vi "SOC_FM Main.vi"() -> ()   [LabVIEW 2015]
doc: "This sample project is built upon the standard state machine template and shows how you could create an application that acquires, analyzes, and presents data. It includes functionality for presenting configuration dialogs, preserving settings between executions, loading and saving data, as well as exporting graph images and text files.\n\nIt is most appropriate for data that is acquired instantly as it does not allow for screen updates mid acquisition nor does it allow for continuous streaming to disk."
uses:
  controls/SOC_FM State.ctl
  controls/SOC_FM Data.ctl
  controls/SOC_FM UI References.ctl
  controls/SOC_FM Graph Data.ctl
  <vilib>/Utility/miscctls.llb/LVAnnotationListTypeDef.ctl
  <vilib>/Utility/miscctls.llb/LVCursorListTypeDef.ctl
  controls/SOC_FM HW Configuration.ctl
  controls/SOC_FM Simulated Signal Type.ctl
  controls/SOC_FM Analysis Configuration.ctl
  controls/SOC_FM New Data Behavior.ctl
  PPL/AbstractCalcLib.lvlibp/AbstractCalc/AbstractCalc.lvclass
  subVIs/SOC_FM Settings Dialog.vi
panel:
  in  "Settings":bool
  in  "Snapshot":bool
  in  "Analyze":bool
  in  "Clear":bool
  in  "Exit":bool
  in  "Acquire":bool
  in  "Export":bool
  in  "Save Data":bool
  in  "Load Data":bool
  out "Graph":waveform(dbl)[](graph)
  out "Status Bar":string
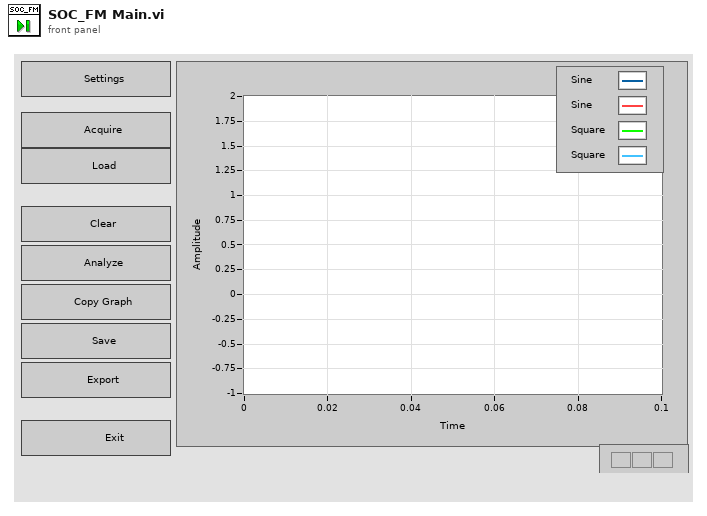
[diagram p1: front panel]
types:
  T1 = typedef "SOC_FM Data.ctl" = cluster{"UI References":T2, "Graph Data":T3, "User Specified":cluster{"Hardware Configuration":T6, "Analysis Configuration":T8, "New Data Behavior":T9, "Calc PPL Path":path, "Calc Plugin Class Qualified Name":string, "Calc Configuration String":string}, "AbstractCalc":refnum<class "AbstractCalc.lvclass">}
  T2 = typedef "SOC_FM UI References.ctl" = cluster{"Exit Ref":refnum<vi>, "Save Ref":refnum<vi>, "Open Ref":refnum<vi>, "Export Ref":refnum<vi>, "Acquire Ref":refnum<vi>, "Configure Ref":refnum<vi>, "Graph Ref":refnum<vi>, "Clear Ref":refnum<vi>, "Analyze Ref":refnum<vi>, "Status Ref":refnum<vi>, "Snapshot Ref":refnum<vi>}
  T3 = typedef "SOC_FM Graph Data.ctl" = cluster{"Data":waveform(dbl)[], "Annotation List":T4, "Cursor List":T5, "Analysis Data":waveform(dbl)[]}
  T4 = typedef "LVAnnotationListTypeDef.ctl" = cluster{"Name":string, "Color":u32, "Style":u8, "Point Style":u8, "Name Visible":bool, "Allow Drag":bool, "Annotation Mode":u32, "Plot":i32, "Index":i32, "Position":cluster{"X":dbl, "Y":dbl}, "X Scale":u32, "Y Scale":u32, "Show Arrow":bool, "Lock Name":bool, "Plot Area":i32, "Label Offset":cluster{"X":dbl, "Y":dbl}}[]
  T5 = typedef "LVCursorListTypeDef.ctl" = cluster{"Name":string, "Color":u32, "Style":u8, "Point Style":u8, "Name Visible":bool, "Allow Drag":bool, "Cursor Mode":u32, "Plot":i32, "Index":i32, "Position":cluster{"X":dbl, "Y":dbl}, "X Scale":u32, "Y Scale":u32, "Watch Plots":i32[], "Watch All Plots":bool, "Plot Area":i32, "Label Offset":cluster{"X":dbl, "Y":dbl}}[]
  T6 = typedef "SOC_FM HW Configuration.ctl" = cluster{"HW Refnum <Replace Me>":string, "Signal Type <Replace Me>":T7}
  T7 = typedef "SOC_FM Simulated Signal Type.ctl" = enum16{"Sine Wave", "Square Wave"}
  T8 = typedef "SOC_FM Analysis Configuration.ctl" = cluster{"Statistics":bool}
  T9 = typedef "SOC_FM New Data Behavior.ctl" = enum16{"Replace", "Overlay", "Append"}
  T10 = typedef "SOC_FM State.ctl" = enum16{"Initialize", "Wait for Event", "Update UI", "Configure", "Acquire", "Load Data", "Save Data", "Clear Data", "Export Data", "Analyze", "Copy Graph", "Exit"}
  T11 = cluster{"Hardware Configuration":T6, "Analysis Configuration":T8, "New Data Behavior":T9, "Calc PPL Path":path, "Calc Plugin Class Qualified Name":string, "Calc Configuration String":string}
  T12 = typedef "SOC_FM User Specified Data.ctl" = cluster{"Hardware Configuration":T6, "Analysis Configuration":T8, "New Data Behavior":T9, "Calc PPL Path":path, "Calc Plugin Class Qualified Name":string, "Calc Configuration String":string}
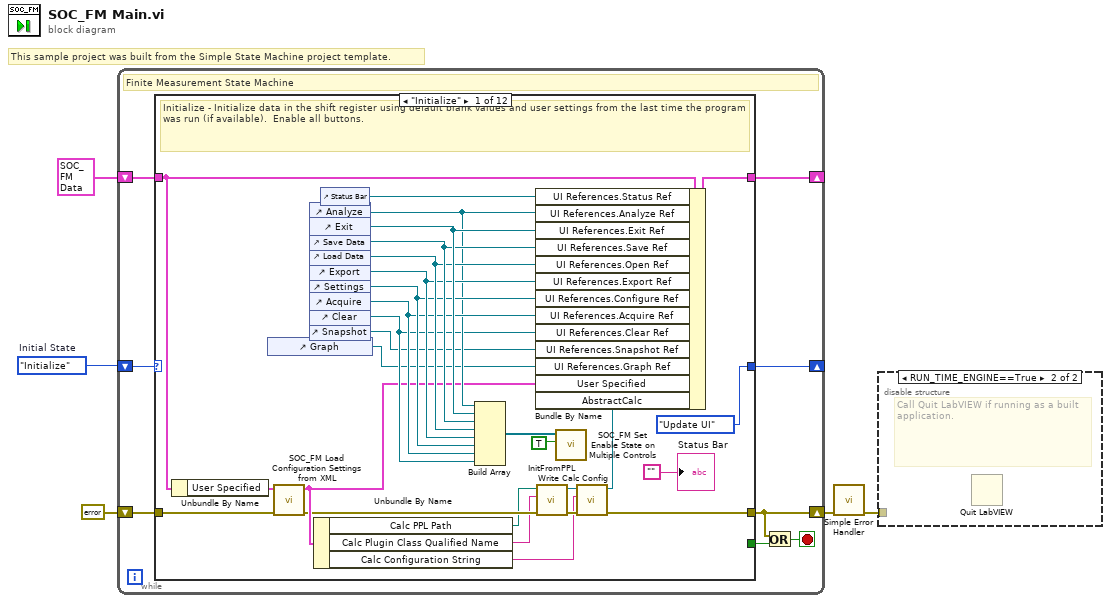
[diagram p0: block diagram]
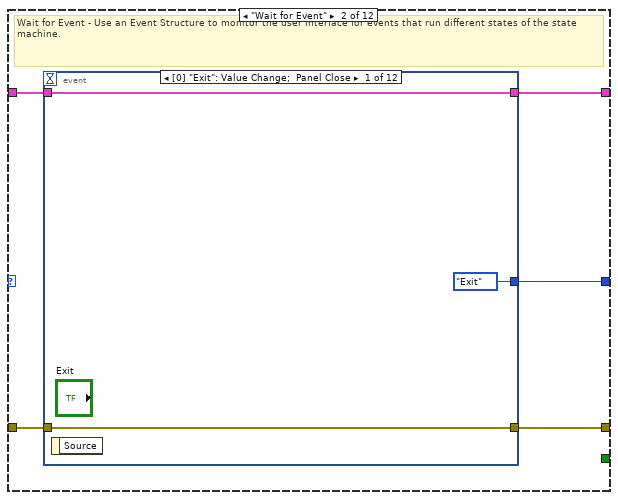
[diagram p3: hidden frame]
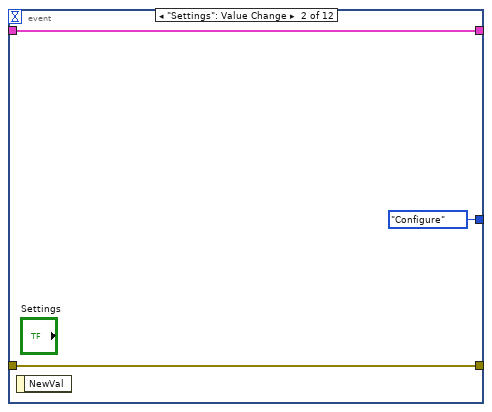
[diagram p4: hidden frame]
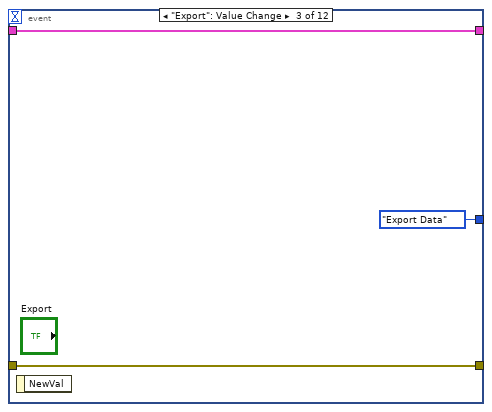
[diagram p5: hidden frame]
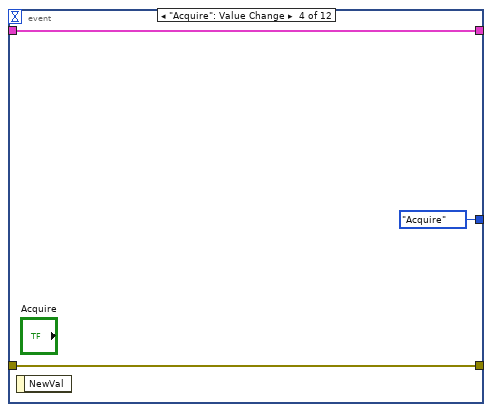
[diagram p6: hidden frame]
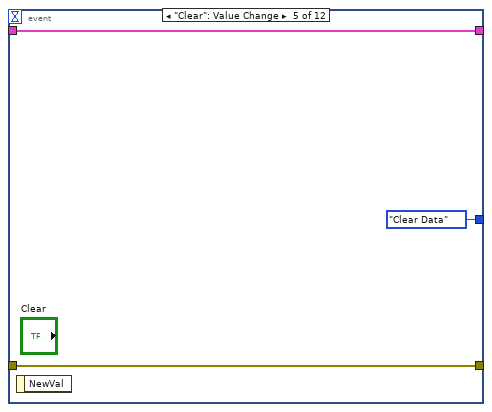
[diagram p7: hidden frame]
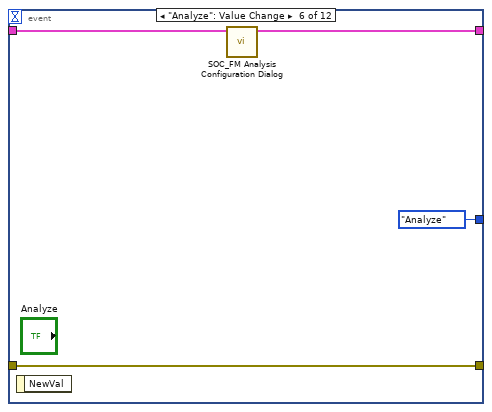
[diagram p8: hidden frame]
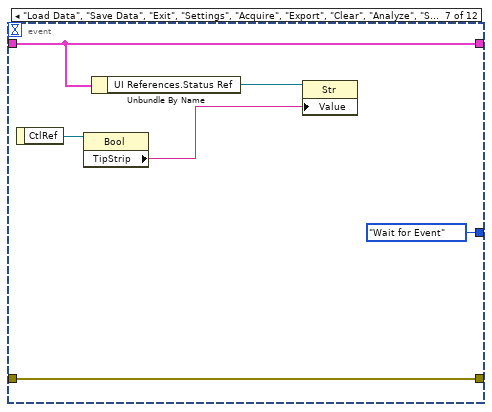
[diagram p9: hidden frame]
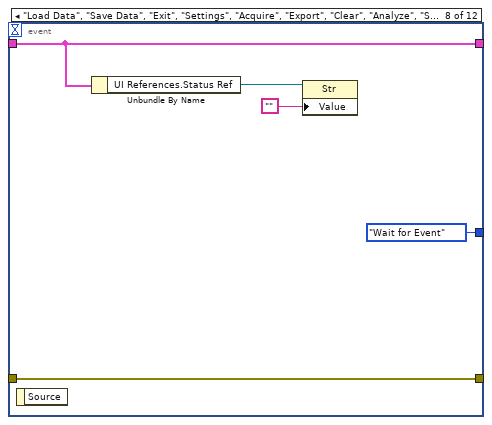
[diagram p10: hidden frame]
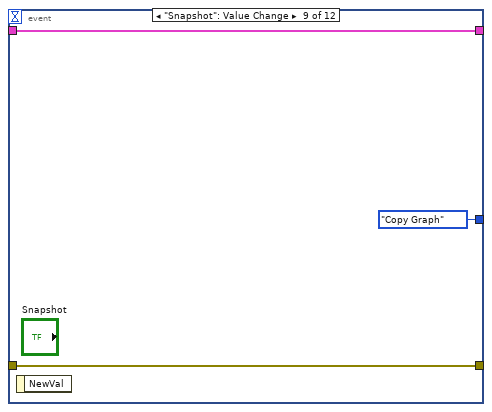
[diagram p11: hidden frame]
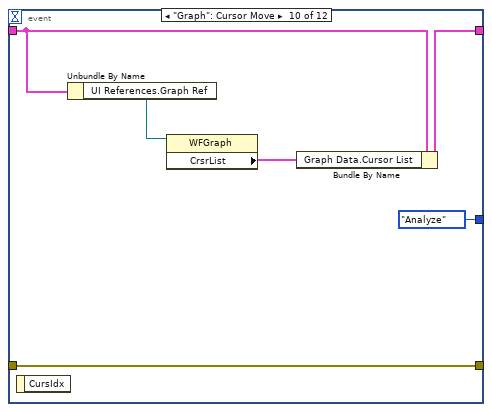
[diagram p12: hidden frame]
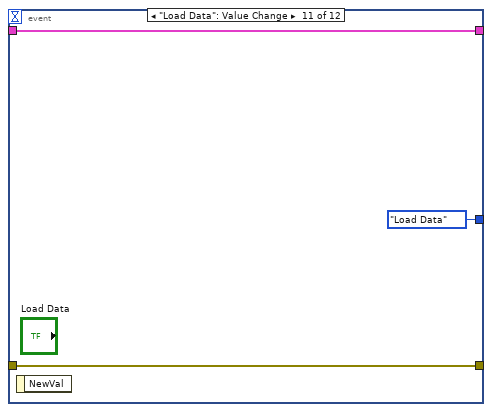
[diagram p13: hidden frame]
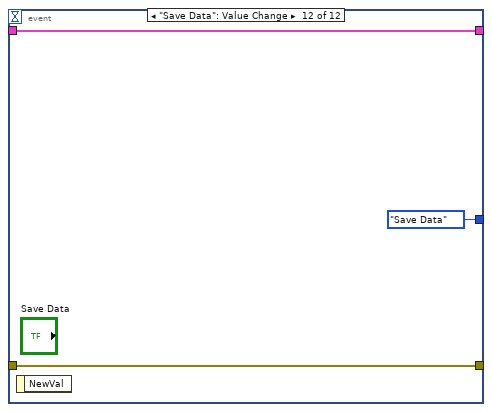
[diagram p14: hidden frame]
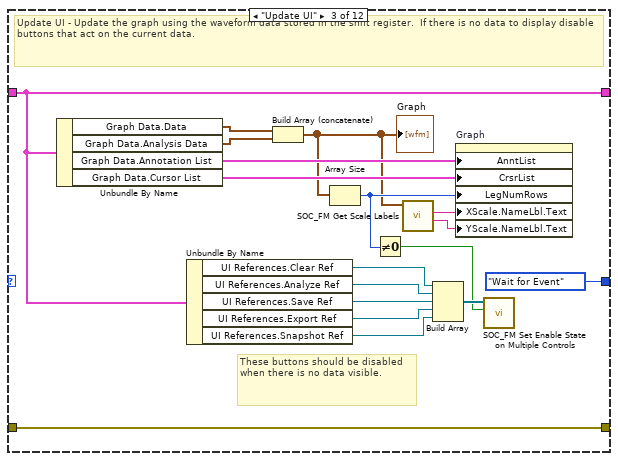
[diagram p15: hidden frame]
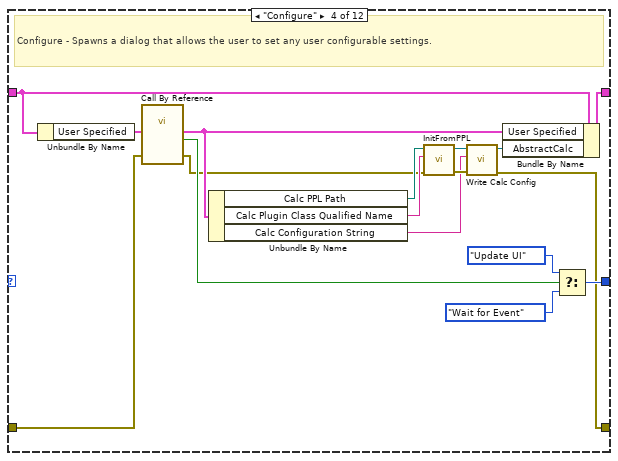
[diagram p16: hidden frame]
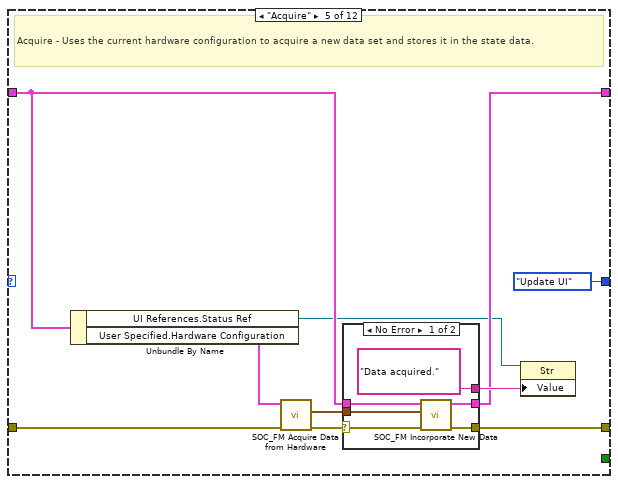
[diagram p17: hidden frame]
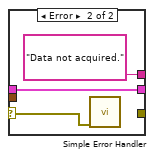
[diagram p18: hidden frame]
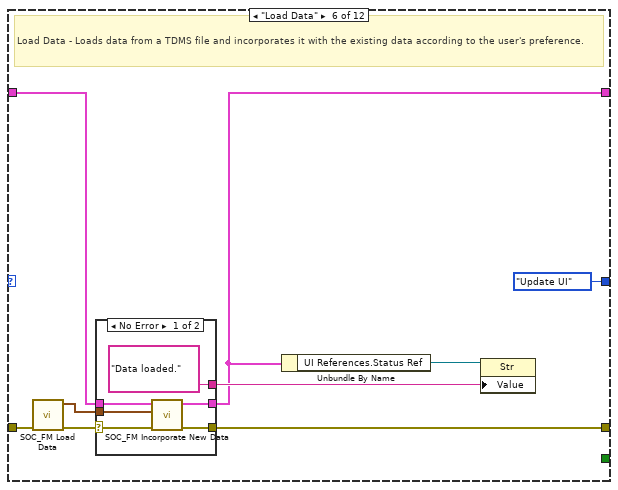
[diagram p19: hidden frame]
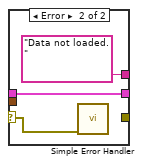
[diagram p20: hidden frame]
diagram:
  w5 = SOC_FM_State."Initialize"  # Initial State
  # "This sample project was built from the Simple State Machine project template."
  n1 = while {
    shift-right: [w12] -> _
    shift-left: w5 -> [w13]
    shift-right: [w10] -> _
    shift-left: T1 {"UI References"={"Exit Ref"=refnum, "Save Ref"=refnum, "Open Ref"=refnum, "Export Ref"=refnum, "Acquire Ref"=refnum, "Configure Ref"=refnum, "Graph Ref"=refnum, "Clear Ref"=refnum, "Analyze Ref"=refnum, "Status Ref"=refnum, "Snapshot Ref"=refnum}, "Graph Data"={"Data"=[], "Annotation List"=[], "Cursor List"=[], "Analysis Data"=[]}, "User Specified"={"Hardware Configuration"={"HW Refnum <Replace Me>"="", "Signal Type <Replace Me>"=enum."Sine Wave"}, "Analysis Configuration"={"Statistics"=TRUE}, "New Data Behavior"=enum."Replace", "Calc PPL Path"=path "", "Calc Plugin Class Qualified Name"="", "Calc Configuration String"=""}, "AbstractCalc"=refnum} ("Data") -> [w11]
    shift-right: [w6] -> w3
    shift-left: errorcluster {"status"=FALSE, "code"=0, "source"=""} ("error constant") -> [w9]
    stop <- w7 stop-if-true
    # "Finite Measurement State Machine"
    n2 = case shown="\"Initialize\"" w13 {
      tunnel: [SOC_FM_State."Update UI" ("Next State") w46 SOC_FM_State."Wait for Event" ("(Value Not Used)") w121 SOC_FM_State."Update UI" ("Next State") SOC_FM_State."Update UI" ("(Value Not Used)") SOC_FM_State."Wait for Event" ("(Value Not Used)") SOC_FM_State."Wait for Event" ("(Value Not Used)") SOC_FM_State."Update UI" ("(Value Not Used)") SOC_FM_State."Update UI" ("(Value Not Used)") SOC_FM_State."Wait for Event" ("(Value Not Used)") w212] -> w12
      tunnel: [_ _ _ _ _ _ _ _ _ _ _ w211] -> w8
      tunnel: w11 -> [w32 w45 w106 w126 w132 w154 w167 w179 w190 w199 w203 w209]
      tunnel: [w40 w44 w106 w125 w131 w148 w167 w179 w189 w199 w203 w209] -> w10
      tunnel: w9 -> [w30 w43 w109 w124 w134 w153 w169 w182 w192 w196 w202 w206]
      tunnel: [w19 w42 w109 w110 w127 w152 w165 w176 w192 w193 w201 w205] -> w6
      frame "Initialize" {
        # "Initialize - Initialize data in the shift register using default blank values and user settings from the last time the program was run (if available).  Enable all buttons."
        n3 = Unbundle By Name(w32) -> ("User Specified"=w31:T11)
        n4 = control-ref of="Graph"() -> (w23:refnum<vi>)
        n5 = call "SOC_FM Load Configuration Settings from XML.vi"("error in (no error)"=w30, "User Specified"=w31) -> ("error out"=w21:errorcluster, "User Specified 2"=w22:T12)  [unwired: 8 in]
        n6 = control-ref of="Analyze"() -> (w29:refnum<vi>)
        n7 = control-ref of="Exit"() -> (w39:refnum<vi>)
        n8 = control-ref of="Save Data"() -> (w38:refnum<vi>)
        n9 = control-ref of="Load Data"() -> (w37:refnum<vi>)
        n10 = control-ref of="Export"() -> (w36:refnum<vi>)
        n11 = control-ref of="Settings"() -> (w35:refnum<vi>)
        n12 = control-ref of="Acquire"() -> (w34:refnum<vi>)
        n13 = control-ref of="Clear"() -> (w27:refnum<vi>)
        n14 = control-ref of="Snapshot"() -> (w24:refnum<vi>)
        n15 = Unbundle By Name(w22) -> ("Calc PPL Path"=w14:path, "Calc Plugin Class Qualified Name"=w15:string, "Calc Configuration String"=w17:string)
        n16 = control-ref of="Status Bar"() -> (w28:refnum<vi>)
        n17 = Build Array(w29, w39, w38, w37, w36, w35, w34, w27) -> (w33:refnum<vi>[])
        n18 = call "InitFromPPL.vi"("error in (no error)"=w21, "qualified name"=w15, "packed library path"=w14) -> ("error out"=w20:errorcluster, "AbstractCalc out"=w16:refnum<class "AbstractCalc.lvclass">)  [unwired: 7 in]
        n19 = call "SOC_FM Set Enable State on Multiple Controls.vi"("Enable?"=TRUE, "Controls"=w33) -> ()  [unwired: 10 in]
        n20 = call-dynamic "Write Calc Config.vi"("error in (no error)"=w20, "Config String"=w17, "AbstractCalc in"=w16) -> ("error out"=w19:errorcluster, "AbstractCalc out"=w18:refnum<class "AbstractCalc.lvclass">)  [unwired: 7 in]
        n21 = Bundle By Name(cluster=w32, "UI References.Status Ref"=w28, "UI References.Analyze Ref"=w29, "UI References.Exit Ref"=w39, "UI References.Save Ref"=w38, "UI References.Open Ref"=w37, "UI References.Export Ref"=w36, "UI References.Configure Ref"=w35, "UI References.Acquire Ref"=w34, "UI References.Clear Ref"=w27, "UI References.Snapshot Ref"=w24, "UI References.Graph Ref"=w23, "User Specified"=w22, "AbstractCalc"=w18) -> (w40:T1)
        "Status Bar" <- "" ("Status Bar")
      }
      frame "Wait for Event" {
        # "Wait for Event - Use an Event Structure to monitor the user interface for events that run different states of the state machine."
        n22 = event shown="[0] \"Exit\": Value Change;  Panel Close" {
          selector: _ -> [_ _ _ _ _ _ _ _ _ _ _ _]
          dyn-events: _ -> [_ _ _ _ _ _ _ _ _ _ _ _]
          timeout: _ -> [_ _ _ _ _ _ _ _ _ _ _ _]
          tunnel: [SOC_FM_State."Exit" ("Next State") SOC_FM_State."Configure" ("Next State") SOC_FM_State."Export Data" ("Next State") SOC_FM_State."Acquire" ("Next State") SOC_FM_State."Clear Data" ("Next State") SOC_FM_State."Analyze" ("Next State") SOC_FM_State."Wait for Event" ("Next State") SOC_FM_State."Wait for Event" ("Next State") SOC_FM_State."Copy Graph" ("Next State") SOC_FM_State."Analyze" ("Next State") SOC_FM_State."Load Data" ("Next State") SOC_FM_State."Save Data" ("Next State")] -> w46
          tunnel: w45 -> [w48 w52 w55 w58 w61 w63 w69 w75 w79 w80 w87 w90]
          tunnel: [w48 w52 w55 w58 w61 w62 w69 w75 w79 w83 w87 w90] -> w44
          tunnel: w43 -> [w47 w51 w54 w57 w60 w65 w71 w76 w78 w85 w86 w89]
          tunnel: [w47 w51 w54 w57 w60 w65 w71 w76 w78 w85 w86 w89] -> w42
          event "Exit": Value Change; Panel Close {
            n23 = event-data() -> ()  [unwired: 1 in, 1 out]
          }
          event "Settings": Value Change {
            n24 = event-data() -> ()  [unwired: 1 in, 1 out]
          }
          event "Export": Value Change {
            n25 = event-data() -> ()  [unwired: 1 in, 1 out]
          }
          event "Acquire": Value Change {
            n26 = event-data() -> ()  [unwired: 1 in, 1 out]
          }
          event "Clear": Value Change {
            n27 = event-data() -> ()  [unwired: 1 in, 1 out]
          }
          event "Analyze": Value Change {
            n28 = event-data() -> ()  [unwired: 1 in, 1 out]
            n29 = call "SOC_FM Analysis Configuration Dialog.vi"("Data"=w63) -> ("Data 2"=w62:T1)  [unwired: 10 in]
          }
          event "Load Data", "Save Data", "Exit", "Settings", "Acquire", "Export", "Clear", "Analyze", "Snapshot": Mouse Enter {
            n30 = event-data() -> ("CtlRef"=w70:refnum<vi>)  [unwired: 1 in]
            n31 = property class="Bool"(reference=w70) -> ("TipStrip"=w67:string)  [unwired: 1 in, 2 out]
            n32 = Unbundle By Name(w69) -> ("UI References.Status Ref"=w68:refnum<vi>)
            n33 = property class="Str"(reference=w68, "Value"=w67) -> ()  [unwired: 1 in, 2 out]
          }
          event "Load Data", "Save Data", "Exit", "Settings", "Acquire", "Export", "Clear", "Analyze", "Snapshot": Mouse Leave {
            n34 = event-data() -> ()  [unwired: 1 in, 1 out]
            n35 = Unbundle By Name(w75) -> ("UI References.Status Ref"=w74:refnum<vi>)
            n36 = property class="Str"(reference=w74, "Value"="") -> ()  [unwired: 1 in, 2 out]
          }
          event "Snapshot": Value Change {
            n37 = event-data() -> ()  [unwired: 1 in, 1 out]
          }
          event "Graph": Cursor Move {
            n38 = event-data() -> ()  [unwired: 1 in, 1 out]
            n39 = Unbundle By Name(w80) -> ("UI References.Graph Ref"=w82:refnum<vi>)
            n40 = property class="WFGraph"(reference=w82) -> ("CrsrList"=w81:T5)  [unwired: 1 in, 2 out]
            n41 = Bundle By Name(cluster=w80, "Graph Data.Cursor List"=w81) -> (w83:T1)
          }
          event "Load Data": Value Change {
            n42 = event-data() -> ()  [unwired: 1 in, 1 out]
          }
          event "Save Data": Value Change {
            n43 = event-data() -> ()  [unwired: 1 in, 1 out]
          }
        }
      }
      frame "Update UI" {
        # "These buttons should be disabled when there is no data visible."
        # "Update UI - Update the graph using the waveform data stored in the shift register.  If there is no data to display disable buttons that act on the current data."
        n44 = Unbundle By Name(w106) -> ("Graph Data.Data"=w102:waveform(dbl)[], "Graph Data.Analysis Data"=w92:waveform(dbl)[], "Graph Data.Annotation List"=w107:T4, "Graph Data.Cursor List"=w103:T5)
        n45 = Unbundle By Name(w106) -> ("UI References.Clear Ref"=w98:refnum<vi>, "UI References.Analyze Ref"=w97:refnum<vi>, "UI References.Save Ref"=w105:refnum<vi>, "UI References.Export Ref"=w95:refnum<vi>, "UI References.Snapshot Ref"=w96:refnum<vi>)
        n46 = Build Array (concatenate)(w102, w92) -> (w100:waveform(dbl)[])
        "Graph" <- w100
        n47 = Array Size(array=w100) -> (size(s)=w101:i32)
        n48 = Not Equal To 0?(x=w101) -> (x != 0?=w99:bool)
        n49 = call "SOC_FM Get Scale Labels.vi"("Array of Waveforms"=w100) -> ("Y Scale Label Text"=w93:string, "X Scale Label Text"=w94:string)  [unwired: 9 in]
        n50 = Build Array(w98, w97, w105, w95, w96) -> (w104:refnum<vi>[])
        n51 = property on="Graph" class="WFGraph (strict)"("AnntList"=w107, "CrsrList"=w103, "LegNumRows"=w101, "XScale.NameLbl.Text"=w94, "YScale.NameLbl.Text"=w93) -> ()  [unwired: 2 in, 2 out]
        n52 = call "SOC_FM Set Enable State on Multiple Controls.vi"("Enable?"=w99, "Controls"=w104) -> ()  [unwired: 10 in]
      }
      frame "Configure" {
        # "Configure - Spawns a dialog that allows the user to set any user configurable settings."
        n53 = Unbundle By Name(w126) -> ("User Specified"=w119:T11)
        n54 = call-by-ref "?"("error in (no error)"=w124, "User Specified"=w119) -> ("error out"=w111:errorcluster, "UI Refresh Needed?"=w123:bool, "User Specified 2"=w117:T12)  [unwired: 9 in, 2 out]
        n55 = Unbundle By Name(w117) -> ("Calc PPL Path"=w114:path, "Calc Plugin Class Qualified Name"=w112:string, "Calc Configuration String"=w113:string)
        n56 = call "InitFromPPL.vi"("error in (no error)"=w111, "qualified name"=w112, "packed library path"=w114) -> ("error out"=w116:errorcluster, "AbstractCalc out"=w118:refnum<class "AbstractCalc.lvclass">)  [unwired: 7 in]
        n57 = call-dynamic "Write Calc Config.vi"("error in (no error)"=w116, "Config String"=w113, "AbstractCalc in"=w118) -> ("error out"=w110:errorcluster, "AbstractCalc out"=w115:refnum<class "AbstractCalc.lvclass">)  [unwired: 7 in]
        n58 = Bundle By Name(cluster=w126, "User Specified"=w117, "AbstractCalc"=w115) -> (w125:T1)
        n59 = Select(t=SOC_FM_State."Update UI" ("Next State if true"), s=w123, f=SOC_FM_State."Wait for Event" ("Next State if false")) -> (s? t:f=w121:T10)
      }
      frame "Acquire" {
        # "Acquire - Uses the current hardware configuration to acquire a new data set and stores it in the state data."
        n60 = Unbundle By Name(w132) -> ("UI References.Status Ref"=w128:refnum<vi>, "User Specified.Hardware Configuration"=w135:T6)
        n61 = call "SOC_FM Acquire Data from Hardware.vi"("error in (no error)"=w134, "Hardware Configuration"=w135) -> ("error out"=w129:errorcluster, "Graph Data"=w130:waveform(dbl)[])  [unwired: 8 in]
        n62 = case shown="No Error" w129 {
          selector: w129 -> [w139 w144]
          tunnel: w132 -> [w138 w145]
          tunnel: [w142 w145] -> w131
          tunnel: [w141 _] -> w127
          tunnel: w130 -> [w140 _]
          tunnel: ["Data acquired." ("Data acquired") "Data not acquired." ("Data not acquired")] -> w133
          frame No Error {
            n63 = call "SOC_FM Incorporate New Data.vi"("error in (no error)"=w139, "New Graph Data"=w140, "Data"=w138) -> ("error out"=w141:errorcluster, "Data 2"=w142:T1)  [unwired: 7 in]
          }
          frame Error {
            n64 = call <vilib>:"Simple Error Handler.vi"("error in (no error)"=w144) -> ()  [unwired: 4 in, 5 out]
          }
        }
        n65 = property class="Str"(reference=w128, "Value"=w133) -> ()  [unwired: 1 in, 2 out]
      }
      frame "Load Data" {
        # "Load Data - Loads data from a TDMS file and incorporates it with the existing data according to the user's preference."
        n66 = call "SOC_FM Load Data.vi"("error in (no error)"=w153) -> ("error out"=w150:errorcluster, "New Graph Data"=w147:waveform(dbl)[])  [unwired: 9 in]
        n67 = case shown="No Error" w150 {
          selector: w150 -> [w157 w162]
          tunnel: w154 -> [w156 w163]
          tunnel: [w160 w163] -> w148
          tunnel: [w159 _] -> w152
          tunnel: w147 -> [w158 _]
          tunnel: ["Data loaded." ("Data loaded") "Data not loaded." ("Data not loaded")] -> w149
          frame No Error {
            n68 = call "SOC_FM Incorporate New Data.vi"("error in (no error)"=w157, "New Graph Data"=w158, "Data"=w156) -> ("error out"=w159:errorcluster, "Data 2"=w160:T1)  [unwired: 7 in]
          }
          frame Error {
            n69 = call <vilib>:"Simple Error Handler.vi"("error in (no error)"=w162) -> ()  [unwired: 4 in, 5 out]
          }
        }
        n70 = Unbundle By Name(w148) -> ("UI References.Status Ref"=w146:refnum<vi>)
        n71 = property class="Str"(reference=w146, "Value"=w149) -> ()  [unwired: 1 in, 2 out]
      }
      frame "Save Data" {
        # "Save Data - Saves the existing measurement data to a TDMS file."
        n72 = Unbundle By Name(w167) -> ("UI References.Status Ref"=w166:refnum<vi>, "Graph Data.Data"=w170:waveform(dbl)[])
        n73 = call "SOC_FM Save Data.vi"("error in (no error)"=w169, "Data"=w170) -> ("error out"=w168:errorcluster)  [unwired: 9 in]
        n74 = case shown="No Error" w168 {
          selector: w168 -> [w172 w175]
          tunnel: ["Data saved." ("Data saved") "Data not saved." ("Data not saved")] -> w164
          tunnel: [w172 _] -> w165
          frame No Error {
          }
          frame Error {
            n75 = call <vilib>:"Simple Error Handler.vi"("error in (no error)"=w175) -> ()  [unwired: 4 in, 5 out]
          }
        }
        n76 = property class="Str"(reference=w166, "Value"=w164) -> ()  [unwired: 1 in, 2 out]
      }
      frame "Export Data" {
        # "Export Data - Exports the currently loaded measurement and analysis data to a text file that can be imported into a spreadsheet or other application."
        n77 = Unbundle By Name(w179) -> ("UI References.Status Ref"=w177:refnum<vi>, "Graph Data"=w178:T3)
        n78 = call "SOC_FM Export Data.vi"("error in (no error)"=w182, "Graph Data"=w178) -> ("error out"=w180:errorcluster)  [unwired: 9 in]
        n79 = case shown="No Error" w180 {
          selector: w180 -> [w184 w187]
          tunnel: ["Data exported." ("Data exported") "Data not exported." ("Data not exported")] -> w181
          tunnel: [w184 _] -> w176
          frame No Error {
          }
          frame Error {
            n80 = call <vilib>:"Simple Error Handler.vi"("error in (no error)"=w187) -> ()  [unwired: 4 in, 5 out]
          }
        }
        n81 = property class="Str"(reference=w177, "Value"=w181) -> ()  [unwired: 1 in, 2 out]
      }
      frame "Clear Data" {
        # "Clear Data - Clears the data currently in the graph."
        n82 = Bundle By Name(cluster=w190, "Graph Data"=T3 {"Data"=[], "Annotation List"=[], "Cursor List"=[], "Analysis Data"=[]} ("Graph")) -> (w189:T1)
      }
      frame "Analyze" {
        # "#CodeRecommended - Create a new class that inherits from AbstractCalc.lvclass."
        # "Analyze - Analyzes the measurement data."
        n83 = Unbundle By Name(w199) -> ("AbstractCalc"=w198:refnum<class "AbstractCalc.lvclass">, "Graph Data.Data"=w197:waveform(dbl)[])
        n84 = call-dynamic "Calc.vi"("error in (no error)"=w196, "ArrayOfWVFMs"=w197, "AbstractCalc in"=w198) -> ("error out"=w194:errorcluster, "Results"=w195:string[])  [unwired: 6 in, 1 out]
        n85 = call "ResultDialog.vi"("error in (no error)"=w194, "Result Array"=w195) -> ("error out"=w193:errorcluster)  [unwired: 9 in]
      }
      frame "Copy Graph" {
        # "Copy Graph - Places an image of the graph on the clipboard for pasting into reports or emails."
        n86 = call "SOC_FM Copy Graph to Clipboard.vi"("error in (no error)"=w202, "Data"=w203) -> ("error out"=w201:errorcluster)  [unwired: 9 in]
      }
      frame "Exit" {
        w211 = TRUE  # Stop Loop?
        w212 = SOC_FM_State."Exit"  # (Value Not Used)
        # "Exit - Saves the user's settings to an XML file and stops execution."
        n87 = Unbundle By Name(w209) -> ("UI References.Status Ref"=w207:refnum<vi>, "User Specified"=w210:T11)
        n88 = call "SOC_FM Save Configuration Settings to XML.vi"("error in (no error)"=w206, "User Specified"=w210) -> ("error out"=w205:errorcluster)  [unwired: 9 in]
        n89 = property class="Str"(reference=w207, "Value"="Application exit." ("Stopped")) -> ()  [unwired: 1 in, 2 out]
      }
    }
    n90 = Or(x=w6, y=w8) -> (x .or. y?=w7:bool)
  }
  n91 = call <vilib>:"Simple Error Handler.vi"("error in (no error)"=w3) -> ("error out"=w1:errorcluster)  [unwired: 4 in, 4 out]
  n92 = disable-structure shown="RUN_TIME_ENGINE==True" {
    disable-tunnel: w1 -> [_ _]
    frame condition #0 (active) {
    }
    frame condition #1 {
      # "Call Quit LabVIEW if running as a built application."
      n93 = Quit LabVIEW() -> ()  [unwired: 1 in]
    }
  }
